vi "GEOM_GUI_getFPA.vi"(10 "name":string) -> (1 "items":i32[](array[numeric]), 2 "fpa info":string[][](array[string]), 4 "readmodes":string[](array[string]), 5 "fpainfo":string)   [LabVIEW 2016]
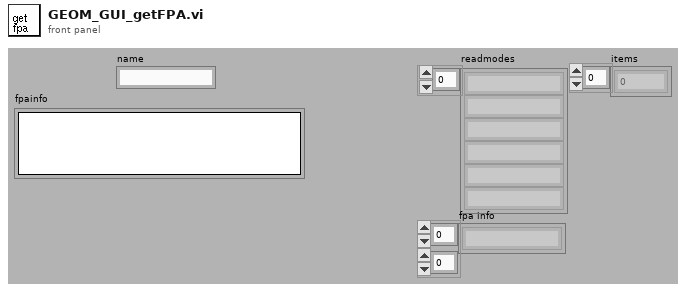
[diagram p1: front panel]
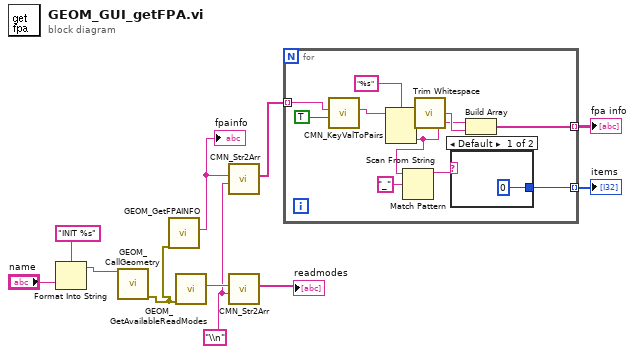
[diagram p0: block diagram]
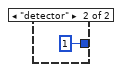
[diagram p2: hidden frame]
diagram:
  w6 = "\\n" ("separator")
  n1 = Format Into String(format string="INIT %s", "name") -> (resulting string=w10:string)  [unwired: 2 in, 1 out]
  n2 = call "GEOM_CallGeometry.vi"("Command"=w10) -> ("error out"=w4:errorcluster)  [unwired: 1 in, 13 out]
  n3 = call "GEOM_GetFPAINFO.vi"("error in (no error)"=w4) -> ("info"=w7:string)  [unwired: 10 out]
  "fpainfo" <- w7
  n4 = call "GEOM_GetAvailableReadModes.vi"("error in (no error)"=w4) -> ("info"=w11:string)  [unwired: 10 out]
  n5 = call "CMN_Str2Arr.vi"("separator"=w6, "string in"=w7) -> ("Array out"=w5:string[])  [unwired: 2 in, 7 out]
  n6 = call "CMN_Str2Arr.vi"("separator"=w6, "string in"=w11) -> ("Array out"=→"readmodes":string[])  [unwired: 2 in, 7 out]
  n7 = for {
    tunnel: w5 -> [w22] mode=indexing
    tunnel: [w16] -> w2 mode=indexing
    tunnel: [w12] -> w1 mode=indexing
    n8 = call "CMN_KeyValToPairs.vi"("replace all? (F)"=TRUE, "key=value pairs"=w22) -> ("arguments out"=w20:string)  [unwired: 9 out]
    n9 = Scan From String(format string="%s", input string=w20) -> (remaining string=w18:string, output 1=w15:string)  [unwired: 2 in, 3 out]
    n10 = Match Pattern(string=w15, regular expression="_") -> (before substring=w13:string)  [unwired: 4 out]
    n11 = call <vilib>:"Trim Whitespace.vi"("string"=w18) -> ("trimmed string"=w17:string)  [unwired: 1 in]
    n12 = case shown="Default" w13 {
      tunnel: [0 1] -> w12
      frame Default {
      }
      frame "detector" {
      }
    }
    n13 = Build Array(w15, w17) -> (w16:string[])
  }
  "fpa info" <- w2
  "items" <- w1
